vi "PXIe-433x Card Page.vi"(8 "error in (no error)":errorcluster, 11 "Node Ptr":T1 format="%.0x") -> (0 "error out":errorcluster)   [LabVIEW 2011, in "PXIe-433x Custom Device.lvlib"]
uses:
  PXIe-433x Custom Device.lvlib
  <vilib>/NI Veristand/Custom Device API/Custom Device Item Ref.ctl
  <vilib>/NI Veristand/Custom Device API/Custom Device API.lvlib
panel:
  in  "Header":cluster{"Section Name":string}={"Section Name"="PXIe-4330 or 4331"}
  in  "Description":string
  in  "Device Name":string
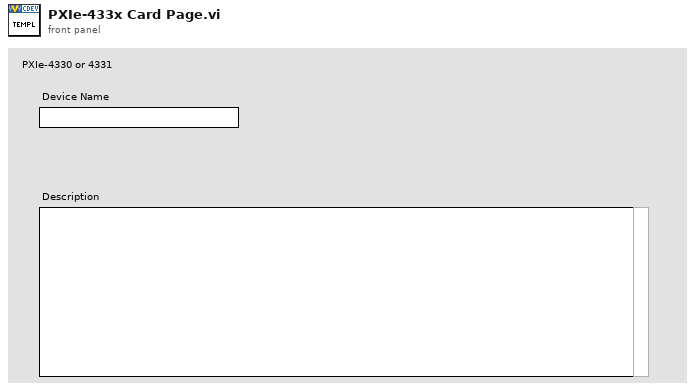
[diagram p1: front panel]
types:
  T1 = typedef "Custom Device API.lvlib/Custom Device Item Ref.ctl" = u64
  T2 = typedef "Custom Device API.lvlib/Custom Device Item Info.ctl" = cluster{"Name":string, "Is Channel":bool, "GUID":string}
  T3 = typedef "Custom Device API.lvlib/Custom Device Commands.ctl" = enum16{"Default", "Item renamed", "Shutdown", "Dynamic button pressed"}
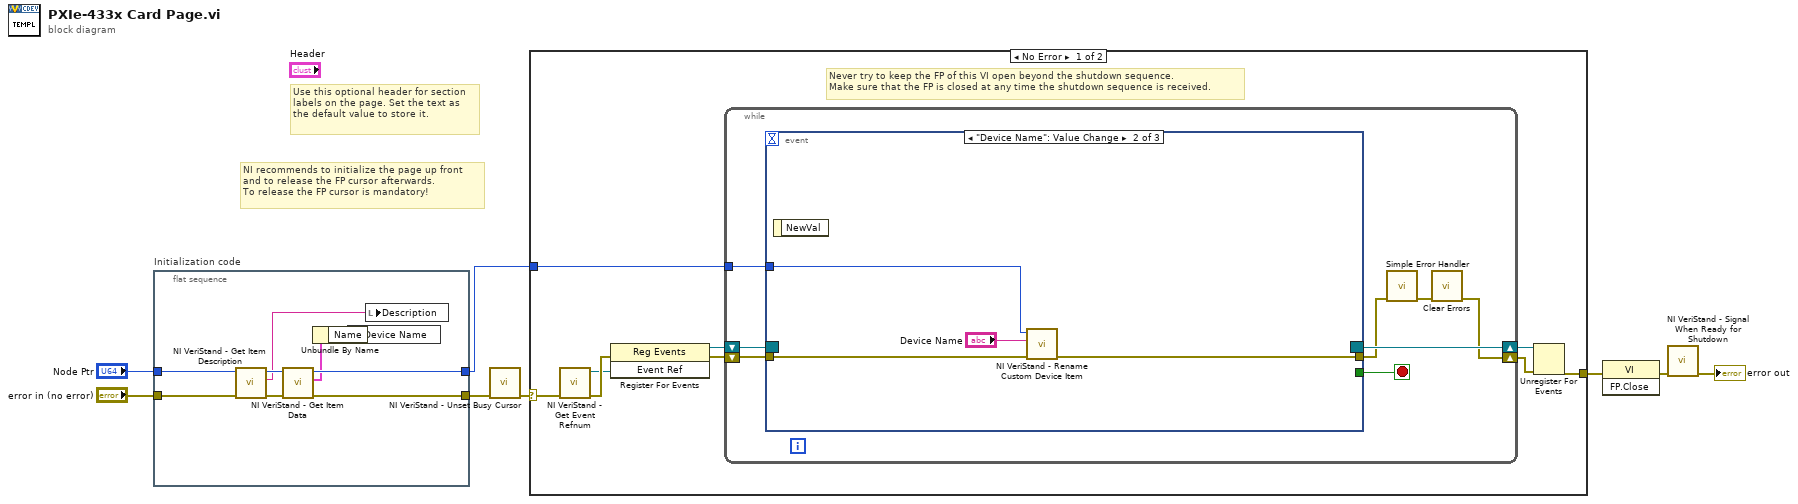
[diagram p0: block diagram]
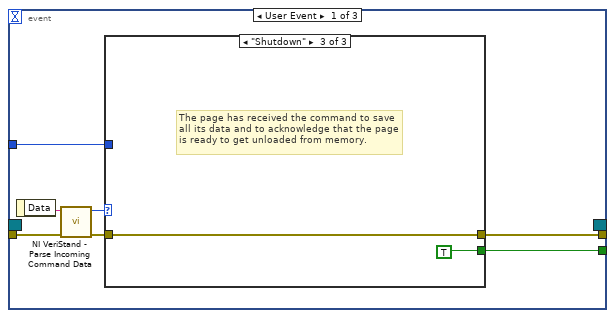
[diagram p2: hidden frame]
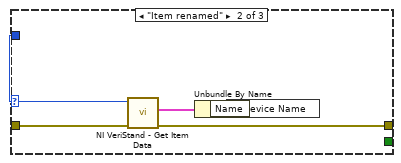
[diagram p4: hidden frame]
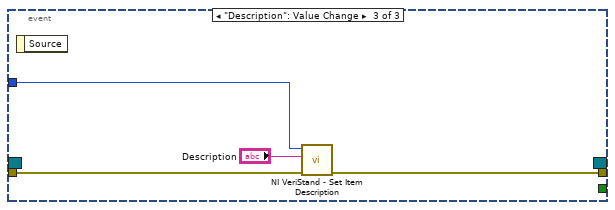
[diagram p5: hidden frame]
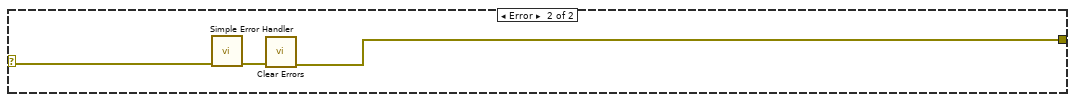
[diagram p6: hidden frame]
diagram:
  # "Use this optional header for section labels on the page. Set the text as the default value to store it."
  # "NI recommends to initialize the page up front\nand to release the FP cursor afterwards.\nTo release the FP cursor is mandatory!"
  n1 = flat-sequence "Initialization code" {
    tunnel: "error in (no error)" -> [w9]
    tunnel: "Node Ptr" -> [w10]
    tunnel: [w11] -> w1
    tunnel: [w17] -> w2
    frame #0 {
      n2 = call <vilib>:"NI VeriStand - Get Item Description.vi"("error in (no error)"=w9, "Item Ref in"=w10) -> ("error out"=w14:errorcluster, "Description"=w15:string, "Item Ref out"=w16:T1)  [unwired: 7 out]
      n3 = call <vilib>:"NI VeriStand - Get Item Data.vi"("error in (no error)"=w14, "Item Ref in"=w16) -> ("error out"=w11:errorcluster, "Item Info"=w13:T2, "Item Ref out"=w17:T1)  [unwired: 7 out]
      n4 = Unbundle By Name(w13) -> ("Name"=w12:string)
      n5 = local write "Device Name"(w12) -> ()
      n6 = local write "Description"(w15) -> ()
    }
  }
  n7 = call <vilib>:"NI VeriStand - Unset Busy Cursor.vi"("error in (no error)"=w1) -> ("error out"=w4:errorcluster)  [unwired: 10 out]
  n8 = case shown="No Error" w4 {
    selector: w4 -> [w18 w60]
    tunnel: [w23 w58] -> w8
    tunnel: w2 -> [w19 _]
    frame No Error {
      # "Never try to keep the FP of this VI open beyond the shutdown sequence.\nMake sure that the FP is closed at any time the shutdown sequence is received."
      n9 = call <vilib>:"NI VeriStand - Get Event Refnum.vi"("error in (no error)"=w18) -> ("error out"=w26:errorcluster, "Event Ref"=w22:refnum<user-event>)  [unwired: 9 out]
      n10 = register-events(error in=w26, w22) -> (reference out=w20:refnum<event-registration>, error out=w21:errorcluster)  [unwired: 1 in]
      n11 = while {
        tunnel: w19 -> [w30]
        shift-right: [w27] -> w24
        shift-left: w21 -> [w33]
        shift-right: [w34] -> w25
        shift-left: w20 -> [w32]
        stop <- w31 stop-if-true
        n12 = event shown="[1] \"Device Name\": Value Change" {
          selector: w32 -> [_ _ _]
          dyn-events: [_ _ _] -> w34
          timeout: _ -> [_ _ _]
          tunnel: w33 -> [w41 w53 w56]
          tunnel: [w37 _ _] -> w31
          tunnel: [w36 w52 w55] -> w29
          tunnel: w30 -> [w35 w51 w57]
          event User Event {
            n13 = event-data() -> ("Data"=w40:string)  [unwired: 1 out]
            n14 = call <vilib>:"NI VeriStand - Parse Incoming Command Data.vi"("error in (no error)"=w41, "Incoming data"=w40) -> ("error out"=w39:errorcluster, "Action"=w38:T3)  [unwired: 8 out]
            n15 = case shown="\"Shutdown\"" w38 {
              tunnel: w39 -> [w42 w47 w48]
              tunnel: [_ _ TRUE] -> w37
              tunnel: [w42 w44 w48] -> w36
              tunnel: w35 -> [_ w46 _]
              frame "Default", Default {
              }
              frame "Item renamed" {
                n16 = call <vilib>:"NI VeriStand - Get Item Data.vi"("error in (no error)"=w47, "Item Ref in"=w46) -> ("error out"=w44:errorcluster, "Item Info"=w45:T2)  [unwired: 8 out]
                n17 = Unbundle By Name(w45) -> ("Name"=w43:string)
                n18 = local write "Device Name"(w43) -> ()
              }
              frame "Shutdown" {
                # "The page has received the command to save all its data and to acknowledge that the page is ready to get unloaded from memory."
              }
            }
          }
          event "Device Name": Value Change {
            n19 = event-data() -> ()  [unwired: 2 out]
            n20 = call <vilib>:"NI VeriStand - Rename Custom Device Item.vi"("error in (no error)"=w53, "New Name"="Device Name", "Item Ref in"=w51) -> ("error out"=w52:errorcluster)  [unwired: 8 out]
          }
          event "Description": Value Change {
            n21 = event-data() -> ()  [unwired: 2 out]
            n22 = call <vilib>:"NI VeriStand - Set Item Description.vi"("error in (no error)"=w56, "Description"="Description", "Item Ref in"=w57) -> ("error out"=w55:errorcluster)  [unwired: 8 out]
          }
        }
        n23 = call <vilib>:"Simple Error Handler.vi"("error in (no error)"=w29) -> ("error out"=w28:errorcluster)  [unwired: 1 in, 7 out]
        n24 = call <vilib>:"Clear Errors.vi"("error in (no error)"=w28) -> ("error out"=w27:errorcluster)  [unwired: 6 out]
      }
      n25 = Unregister For Events(event registration refnum=w25, error in=w24) -> (error out=w23:errorcluster)
    }
    frame Error {
      n26 = call <vilib>:"Simple Error Handler.vi"("error in (no error)"=w60) -> ("error out"=w59:errorcluster)  [unwired: 1 in, 7 out]
      n27 = call <vilib>:"Clear Errors.vi"("error in (no error)"=w59) -> ("error out"=w58:errorcluster)  [unwired: 6 out]
    }
  }
  n28 = invoke class="VI" method="FP.Close"(error in=w8) -> (error out=w7:errorcluster)  [unwired: 2 in, 2 out]
  n29 = call <vilib>:"NI VeriStand - Signal When Ready for Shutdown.vi"("error in (no error)"=w7) -> ("error out"=→"error out":errorcluster)  [unwired: 10 out]
